vi "流程文件XML解析.vi"(10 "添加的路径":path, 11 "参数簇":T2={"启动参数"=1, "启动模式"=enum."跨度核查", "量程"=enum."低量程"} {"启动参数" items=["总磷"=1, "总氮"=2, "氨氮"=3]}) -> (3 "数组":T1(array[cluster]))   [LabVIEW 2016, in "斯坦道氨氮.lvlib"]
uses:
  <vilib>/xml/Load XML File.vi
  <vilib>/xml/Close Reference(Node).vi
  <resource>/objmgr/DOMUserDefRef.rc
  <vilib>/xml/NI_XML.lvlib
panel:
  out "大小":i32
  out "XML字符串":string="<?xml version=\"1.0\" encoding=\"ISO-8859-1\"?>\n<bookstore>\n<book ISBN=\"978-0545128285\">\n  <title lang=\"en\">The Tales of Beedle the Bard</title>\n  <author>J. K. Rowling</author>\n  <year>2008</year>\n  <price>12.99</price>\n</book>\n<book ISBN=\"978-0316160209\">\n  <title lang=\"en\">Eclipse</title>\n  <author>Stephenie Meyer</author>\n  <year>2007</year>\n  <price>19.99</price>\n</book>\n<book ISBN=\"978-0316067928\">\n  <title lang=\"en\">Breaking Dawn</title>\n  <author>Stephenie Meyer</author>\n  <year>2008</year>\n  <price>22.99</price>\n</book>\n<book ISBN=\"978-0316017923\">\n  <title lang=\"en\">Outliers: The Story of Success</title>\n  <author>Malcolm Gladwell</author>\n  <year>2008</year>\n  <price>27.99</price>\n</book>\n<book ISBN=\"978-0596007645\">\n  <title lang=\"en\">XML in a Nutshell</title>\n  <author>Elliotte Rusty Harold</author>\n  <author>W. Scott Means</author>\n  <year>2004</year>\n  <price>39.95</price>\n</book>\n</bookstore>"
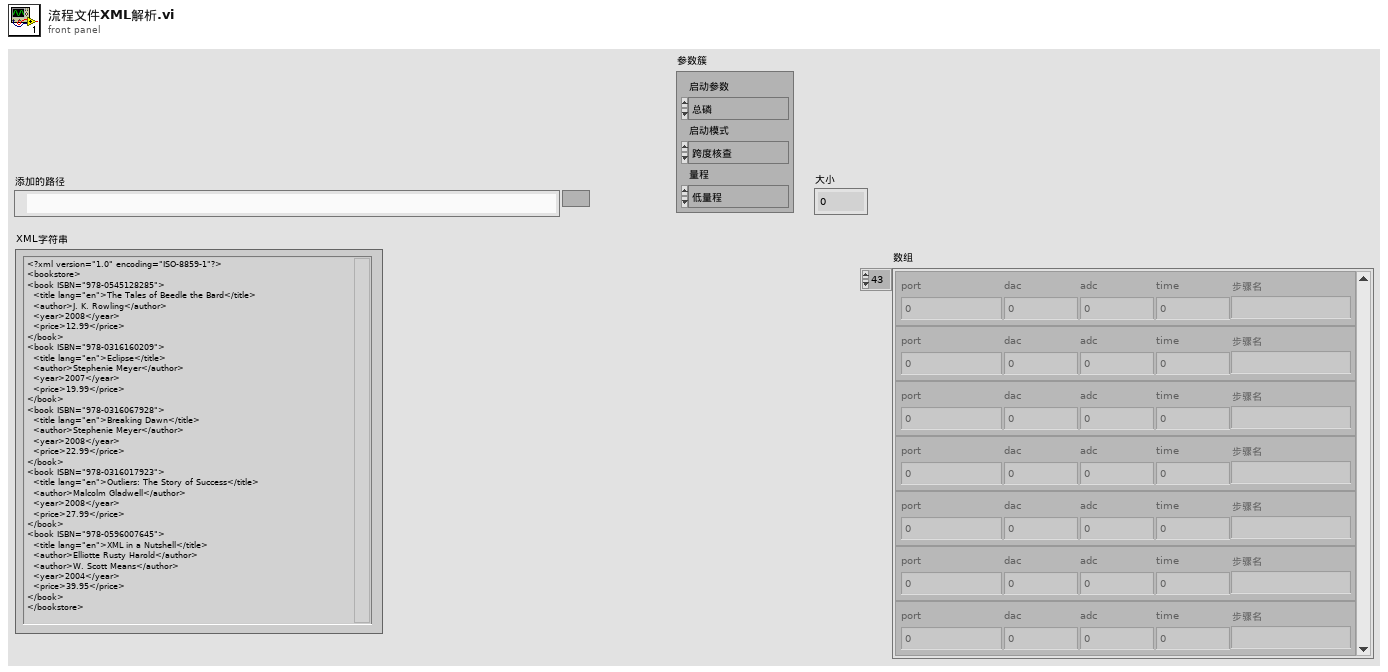
[diagram p1: front panel]
types:
  T1 = cluster{"port":u32, "dac":u8, "adc":u8, "time":u16, "步骤名":string}[]
  T2 = cluster{"启动参数":u16, "启动模式":enum16{"跨度核查", "水样测量", "零点核查", "标样核查", "加标回收"}, "量程":enum16{"低量程", "高量程"}}
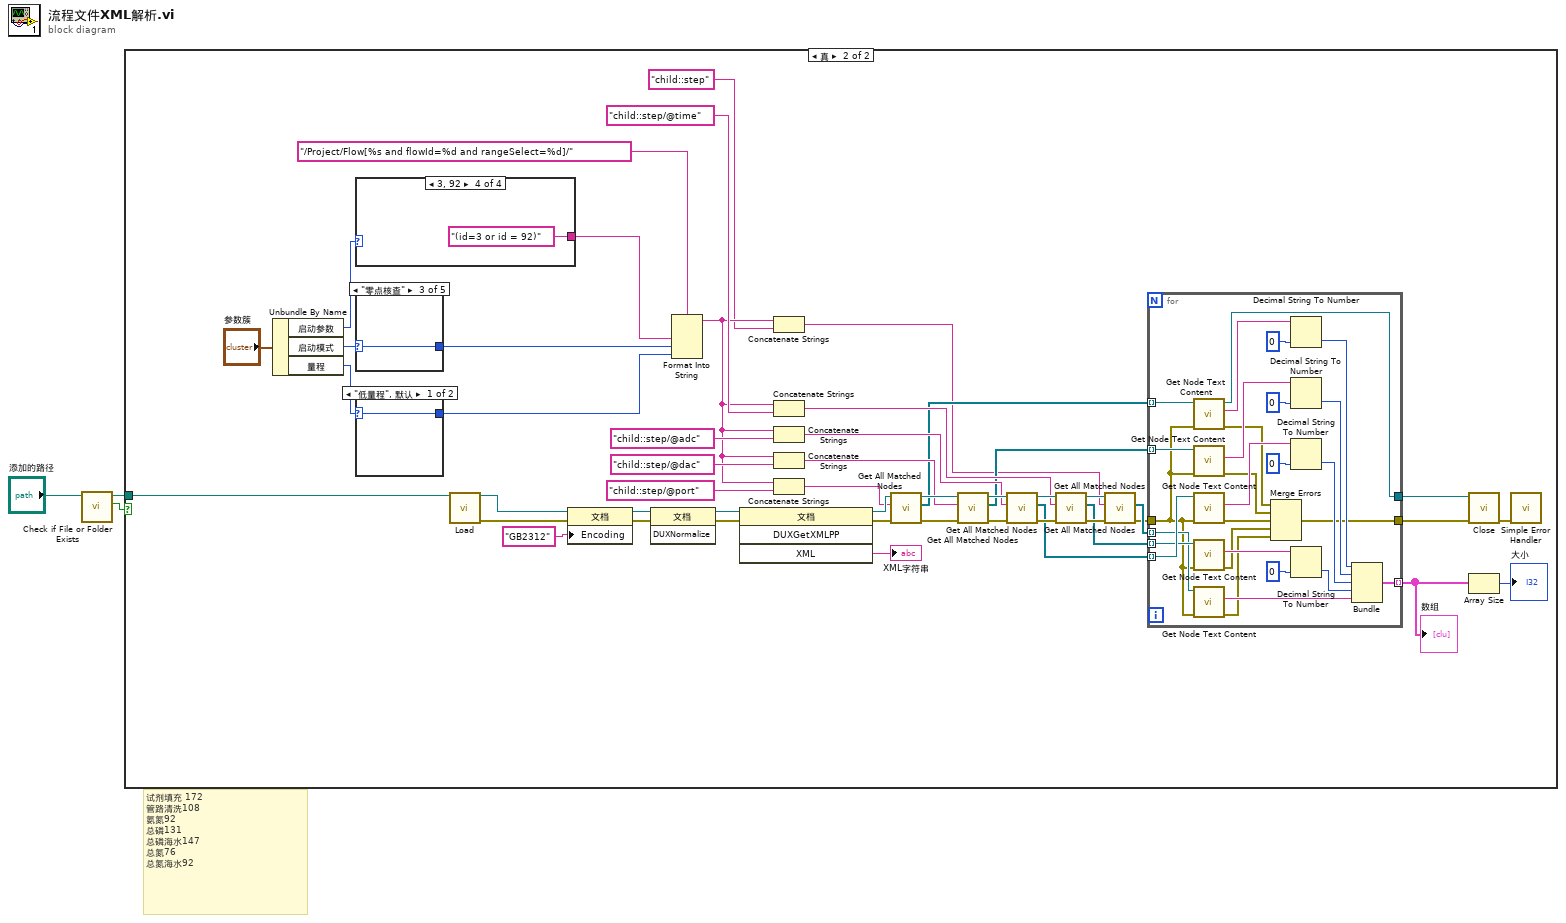
[diagram p0: block diagram]
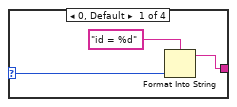
[diagram p3: hidden frame]
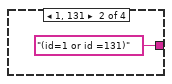
[diagram p4: hidden frame]
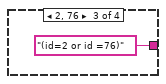
[diagram p5: hidden frame]
diagram:
  # "试剂填充 172 \n管路清洗108\n氨氮92\n总磷131\n总磷海水147\n总氮76\n总氮海水92"
  n1 = call <vilib>:"Check if File or Folder Exists.vi"("path"="添加的路径") -> ("file or folder exists?"=w1:bool, "dup path"=w2:path)  [unwired: 8 in, 1 out]
  n2 = case shown="真" w1 {
    tunnel: w2 -> [_ w34]
    frame False {
    }
    frame True {
      n3 = Unbundle By Name("参数簇") -> ("启动参数"=w36:u16, "启动模式"=w39:enum16{"跨度核查", "水样测量", "零点核查", "标样核查", "加标回收"}, "量程"=w38:enum16{"低量程", "高量程"})
      n4 = case shown="3, 92" w36 {
        selector: w36 -> [w81 _ _ _]
        tunnel: [w80 "(id=1 or id =131)" ("输入 4") "(id=2 or id =76)" ("输入 4") "(id=3 or id = 92)" ("输入 4")] -> w35
        frame 0, Default {
          n5 = Format Into String(format string="id = %d" ("格式字符串"), w81) -> (resulting string=w80:string)  [unwired: 2 in, 1 out]
        }
        frame 1, 131 {
        }
        frame 2, 76 {
        }
        frame 3, 92 {
        }
      }
      n6 = case shown="\"零点核查\"" w39 {
        selector: w39 -> [w88 w89 w90 w91 w92]
        tunnel: [w88 w89 w90 w91 w92] -> w43
        frame "跨度核查", Default {
        }
        frame "水样测量" {
        }
        frame "零点核查" {
        }
        frame "标样核查" {
        }
        frame "加标回收" {
        }
      }
      n7 = case shown="\"低量程\", 默认" w38 {
        selector: w38 -> [w86 w87]
        tunnel: [w86 w87] -> w42
        frame "低量程", Default {
        }
        frame "高量程" {
        }
      }
      n8 = call-poly <vilib>:"Load.vi"("path to XML document"=w34) -> ("DOM document out"=w50:refnum<k20>, "error out"=w49:errorcluster)  [unwired: 12 in, 1 out]
      n9 = property on="属性节点" class="文档"(reference=w50, error in=w49, "Encoding"="GB2312" ("文档编码")) -> (reference out=w48:refnum<k20>, error out=w47:errorcluster)
      n10 = invoke on="Invoke Node" class="文档" method="DUXNormalize"(reference=w48, error in=w47) -> (reference out=w45:refnum<k20>, error out=w46:errorcluster)  [unwired: 1 in, 1 out]
      n11 = Format Into String(format string="/Project/Flow[%s and flowId=%d and rangeSelect=%d]/" ("XPath expression"), w35, w43, w42) -> (resulting string=w16:string)  [unwired: 2 in, 1 out]
      n12 = invoke on="Invoke Node" class="文档" method="DUXGetXMLPP"(reference=w45, error in=w46) -> (reference out=w33:refnum<k20>, error out=w7:errorcluster, "XML"=→"XML字符串":string)  [unwired: 2 in, 1 out]
      n13 = Concatenate Strings(w16, "child::step" ("输入 4")) -> (w9:string)
      n14 = Concatenate Strings(w16, "child::step/@time" ("输入 4")) -> (w18:string)
      n15 = Concatenate Strings(w16, "child::step/@adc" ("输入 4")) -> (w20:string)
      n16 = Concatenate Strings(w16, "child::step/@dac" ("输入 4")) -> (w22:string)
      n17 = Concatenate Strings(w16, "child::step/@port" ("输入 4")) -> (w32:string)
      n18 = call <vilib>:"Get All Matched Nodes.vi"("error in (no error)"=w7, "XPath expression"=w32, "node in"=w33) -> ("error out"=w29:errorcluster, "node result array"=w14:refnum<k20>[], "node out"=w30:refnum<k20>)  [unwired: 6 in]
      n19 = call <vilib>:"Get All Matched Nodes.vi"("error in (no error)"=w29, "XPath expression"=w22, "node in"=w30) -> ("error out"=w28:errorcluster, "node result array"=w13:refnum<k20>[], "node out"=w27:refnum<k20>)  [unwired: 6 in]
      n20 = call <vilib>:"Get All Matched Nodes.vi"("error in (no error)"=w28, "XPath expression"=w20, "node in"=w27) -> ("error out"=w26:errorcluster, "node result array"=w12:refnum<k20>[], "node out"=w25:refnum<k20>)  [unwired: 6 in]
      n21 = call <vilib>:"Get All Matched Nodes.vi"("error in (no error)"=w26, "XPath expression"=w18, "node in"=w25) -> ("error out"=w24:errorcluster, "node result array"=w11:refnum<k20>[], "node out"=w23:refnum<k20>)  [unwired: 6 in]
      n22 = call <vilib>:"Get All Matched Nodes.vi"("error in (no error)"=w24, "XPath expression"=w9, "node in"=w23) -> ("error out"=w8:errorcluster, "node result array"=w10:refnum<k20>[])  [unwired: 6 in, 1 out]
      n23 = for {
        tunnel: w14 -> [w79] mode=indexing
        tunnel: w13 -> [w78] mode=indexing
        tunnel: w12 -> [w77] mode=indexing
        tunnel: w11 -> [w76] mode=indexing
        tunnel: w10 -> [w75] mode=indexing
        tunnel: [w61] -> w4 mode=indexing
        tunnel: w8 -> [w55]
        tunnel: [w54] -> w6
        tunnel: [w53] -> w5
        n24 = call <vilib>:"Get Node Text Content.vi"("error in (no error)"=w55, "node in"=w79) -> ("error out"=w60:errorcluster, "node text"=w74:string, "node out"=w53:refnum<k20>)  [unwired: 7 in]
        n25 = call <vilib>:"Get Node Text Content.vi"("error in (no error)"=w55, "node in"=w78) -> ("error out"=w59:errorcluster, "node text"=w71:string)  [unwired: 7 in, 1 out]
        n26 = call <vilib>:"Get Node Text Content.vi"("error in (no error)"=w55, "node in"=w77) -> ("error out"=w58:errorcluster, "node text"=w68:string)  [unwired: 7 in, 1 out]
        n27 = call <vilib>:"Get Node Text Content.vi"("error in (no error)"=w55, "node in"=w76) -> ("error out"=w57:errorcluster, "node text"=w67:string)  [unwired: 7 in, 1 out]
        n28 = call <vilib>:"Get Node Text Content.vi"("error in (no error)"=w55, "node in"=w75) -> ("error out"=w56:errorcluster, "node text"=w62:string)  [unwired: 7 in, 1 out]
        n29 = Merge Errors(w60, w59, w58, w57, w56) -> (w54:errorcluster)
        n30 = Decimal String To Number(string=w74, default (0L)=u32 0 ("默认(0 I32)")) -> (number=w66:u32)  [unwired: 1 in, 1 out]
        n31 = Decimal String To Number(string=w71, default (0L)=u8 0 ("默认(0 I32)")) -> (number=w65:u8)  [unwired: 1 in, 1 out]
        n32 = Decimal String To Number(string=w68, default (0L)=u8 0 ("默认(0 I32)")) -> (number=w64:u8)  [unwired: 1 in, 1 out]
        n33 = Decimal String To Number(string=w67, default (0L)=u16 0 ("默认(0 I32)")) -> (number=w63:u16)  [unwired: 1 in, 1 out]
        n34 = Bundle(w66, w65, w64, w63, "node text"=w62) -> (w61:cluster{u32, u8, u8, u16, "node text":string})  [unwired: 1 in]
      }
      "数组" <- w4
      n35 = call-poly <vilib>:"Close.vi"("error in (no error)"=w6, "node"=w5) -> ("error out"=w41:errorcluster)  [unwired: 7 out]
      n36 = Array Size(array=w4) -> (size(s)=→"大小":i32)
      n37 = call <vilib>:"Simple Error Handler.vi"("error in (no error)"=w41) -> ()  [unwired: 4 in, 5 out]
    }
  }
